vi "Save Data.vi"(8 "error in (no error)":errorcluster, 11 "Red Pitaya Digitizer in":refnum<class "Red Pitaya Digitizer.lvclass">) -> (0 "error out":errorcluster, 1 "Finished":bool, 2 "Current read position":i32, 3 "Red Pitaya Digitizer out":refnum<class "Red Pitaya Digitizer.lvclass">)   [LabVIEW 2016, in "Red Pitaya Digitizer.lvclass"]
uses:
  Red Pitaya Digitizer.lvclass
  C:/github/NHMFL_Core/Libraries/Instruments/Pulse Driver/Pulse Driver.lvclass
  Red Pitaya Digitizer.lvclass/Red Pitaya Digitizer.ctl
  Instruments/Pulse Driver/Pulse Driver.lvclass/Pulse Driver.ctl
  Read RP Instrument.vi
  Instruments/Pulse Driver/Read Pretrigger samples.vi
  Instruments/Pulse Driver/Read Samples per channel.vi
  Instruments/Pulse Driver/Read Current read position.vi
  Write RP Instrument.vi
  RP Core/RP Instrument/RP Instrument.lvclass
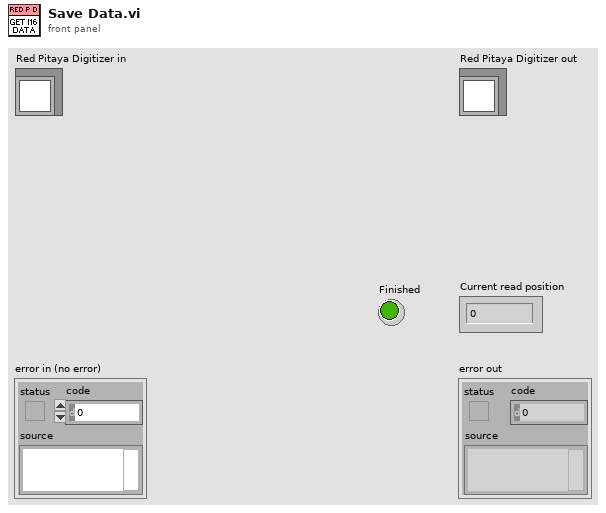
[diagram p1: front panel]
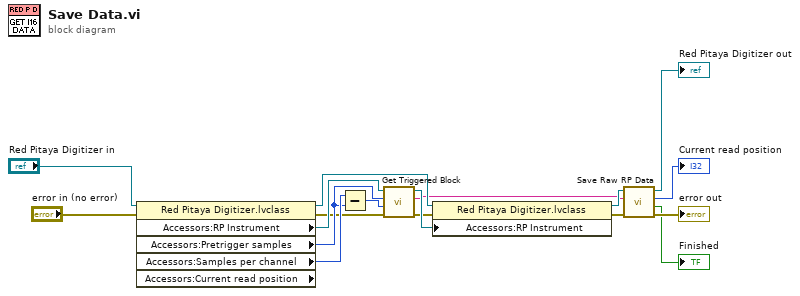
[diagram p0: block diagram]
diagram:
  n1 = property class="Red Pitaya Digitizer.lvclass" props=["Accessors:RP Instrument", "Accessors:Pretrigger samples", "Accessors:Samples per channel", "Accessors:Current read position"](reference="Red Pitaya Digitizer in", error in="error in (no error)") -> (reference out=w16:refnum<class "Red Pitaya Digitizer.lvclass">, error out=w10:errorcluster, "Accessors:RP Instrument"=w14:refnum<class "RP Instrument.lvclass">, "Accessors:Pretrigger samples"=w12:u32, "Accessors:Samples per channel"=w13:i32)  [unwired: 1 out]
  n2 = Subtract(x=w13, y=w12) -> (x-y=w11:u32)
  n3 = call-dynamic "Get Triggered Block.vi"("error in (no error)"=w10, "Post-trigger points"=w11, "Pre-trigger points"=w12, "RP Instrument in"=w14) -> ("error out"=w8:errorcluster, "Data out"=w3:string, "RP Instrument out"=w9:refnum<class "RP Instrument.lvclass">)  [unwired: 5 in]
  n4 = property class="Red Pitaya Digitizer.lvclass"(reference=w16, error in=w8, "Accessors:RP Instrument"=w9) -> (reference out=w7:refnum<class "Red Pitaya Digitizer.lvclass">, error out=w5:errorcluster)
  n5 = call-dynamic "Save Raw RP Data.vi"("error in (no error)"=w5, "Raw data"=w3, "Red Pitaya Digitizer in"=w7) -> ("error out"=→"error out":errorcluster, "Finished"=→"Finished":bool, "Current read position"=→"Current read position":i32, "Red Pitaya Digitizer out"=→"Red Pitaya Digitizer out":refnum<class "Red Pitaya Digitizer.lvclass">)  [unwired: 5 in]
